vi "Locking_using_Photoacoustic_signal_usingcrorrected_intercept_2_custom_locking_with_runningavg_power.vi"() -> ()   [LabVIEW 2021]
uses:
  <vilib>/userDefined/High Color/IMAQdx.ctl
  <vilib>/Analysis/coordinate.llb/2D Cartesian Coordinate Rotation (Array).vi
  <vilib>/Analysis/6fits.llb/Confidence Interval (Linear).vi
  <vilib>/Instr/_visa.llb/VISA Configure Serial Port (Instr).vi
  <vilib>/Analysis/3filter.llb/Zero Phase Filter (DBL).vi
  <vilib>/Analysis/3filter.llb/Butterworth Filter (DBL).vi
  <vilib>/Utility/file.llb/Write Delimited Spreadsheet (DBL).vi
  <vilib>/vision/driver/NI_Vision_Acquisition_Software.lvlib
  <resource>/objmgr/imaqdx.rc
  <vilib>/Analysis/NI_AALBase.lvlib
  <vilib>/Analysis/NI_AAL_SigProc.lvlib
  <vilib>/Analysis/NI_AALPro.lvlib
  <vilib>/ptbypt/NI_PtbyPt.lvlib
  <vilib>/vision/NI_Vision_Development_Module.lvlib
  <instrlib>/Tektronix TBS 2000 Series/Tektronix TBS 2000 Series.lvlib
panel:
  out "Power normalized PAS CH1 2":dbl[](graph)
  out "mean 2":dbl format="%0.5f"
  out "PAS Mean":dbl format="%0.5f"
  out "Initaial value power":dbl format="%#_13g"
  out "mean":dbl format="%0.2f"
  out "millisecond timer value":u32
  in  "Avg Forpower meter":i32
  out "second pass wl 3":dbl format="%#_9g"
  in  "Number of Averages (16) 3":i32=8
  out "Number of Averages (16) 2":i32(ring)=8 items=["2"=2, "4"=4, "8"=8, "16"=16, "32"=32, "64"=64, "128"=128, "256"=256, "512"=512]
  in  "stop":bool
  out "PAS array":dbl[](array[numeric])
  in  "Running averaged power 2":bool
  out "Power(mJ) 2":dbl
  out "source 2":string
  out "Power Measurement with running average2":dbl[](graph)
  out "Normalized PAS 2":dbl format="%#_8g"
  out "Running avg power 2":dbl
  out "horzontal intercept 2":cluster{dbl[], dbl[]}(graph)
  out "Feedback sign 2":dbl
  out "Running avg power":dbl
  out "second pass wl 5":dbl format="%#_9g"
  out "PAS (Process value) 2":dbl format="%#_8g"
  in  "?":T1(tab)
  out "vertical Fringes 2":dbl[](graph)
  out "Horizontal Fringes 2":dbl[](graph)
  out "error out 11":errorcluster
  in  "thor wedge spacing 2":dbl=4.997771500000001 step=1e-06 format="%#_13g"
  out "known wavelength 2":dbl
  out "known wl 2":dbl[](array[numeric])=[591.188, 591.588, 591.988, 592.388, 592.788, 593.188]
  out "obseved wl 2":dbl[](array[numeric])=[591.1849, 591.5523, 591.984, 592.366, 592.7809, 593.169]
  out "Array 7":dbl[](array[numeric])
  out "error out 10":errorcluster
  out "Y Resolution 2":i32
  out "X Resolution 2":i32
  out "initila array horz. fringe 3":ext[](array[numeric])
  out "standard deviation 2":dbl format="%0.5f"
  out "observed wavelength 2":dbl
  out "horz.slope 3":dbl format="%#_7g"
  out "horz.intercept 2":dbl format="%#_8g"
  out "vert intercept 5":dbl
  out "vrt. slope 3":dbl format="%#_9g"
  out "x > y? 2":bool
  out "Locations 2":dbl[](array[numeric])
  in  "vert width 2":i32=5 min=3
  out "hor. std dev 2":dbl format="%0.5f"
  in  "horz. fringe width 2":i32=6 min=3
  in  "wedge angle of thor wedge 3":dbl=0.004681980000000043 format="%#_13g"
  in  "order 6":i32=1
  in  "order 5":i32=2
  out "d value 2":dbl format="%#_10e"
  out "vert.wl 2":dbl
  out "intercept 2":dbl
  out "vert wavelength 2":cluster{dbl[], dbl[]}(graph)
  out "horz intercept value 2":dbl[](array[numeric])
  out "Verticle slope":cluster{dbl[], dbl[]}(graph)
  in  "dimension size":i32=10
  in  "element 3":dbl=0.1 format="%#_15g"
  in  "dimension size 2":i32=10
  in  "element 2":dbl=0.1 format="%#_15g"
  out "vert inteer":dbl[](array[numeric])
  out "Loop time (ms) 2":u32
  out "Array 6":dbl[](array[numeric])
  out "Array 5":ext[](array[numeric])
  out "Buffer Number Out 2":u32
  in  "saturation 3":u32(slide) scale=0.0..128.0
  in  "Gain 3":u32(slide)=1 scale=1.0..128.0
  in  "exposure 3":ext(slide)=0.5 scale=0.0..0.5 scale format="%#_12g"
  out "EnumStrings[] 2":string[](array[string])
  in  "contrast 3":ext(slide)=0.5 scale=0.0..0.5 scale format="%#_12g"
  in  "camera property 2":bool
  in  "index 12":i32=90
  in  "length 11":i32=660
  in  "index 11":i32=400
  in  "length 10":i32=501
  out "horizontal fringe 3":dbl[][](graph)
  in  "index 10":i32=30
  in  "vert-vertical_array length":i32=850
  in  "index 9":i32=500
  in  "length 9":i32=1112
  in  "Slide":dbl(slide)=-2.6530612244897958
  out "VERT FRINGE":dbl[][](graph)
  out "x-y 2":ext
  in  "CONTRAST CUTT OFF VALUE":ext=0.015 format="%#_13g"
  out "initial array vert.  fringe 2":ext[](array[numeric])
  out "Meter":dbl(knob) scale=0.02..0.1 scale format="%#_4g"
  in  "Slide 4":dbl(slide)=-10.204081632653061
  out "count 3":dbl
  out "initial time 2":u32
  out "initial array vert 2":ext[](array[numeric])
  out "initial array horz 3":ext[](array[numeric])
  in  "Tab Control 2":enum32{"real time wavelength measurement"}(tab)
  out "Vertical intercept vs real time":cluster{dbl[], dbl[]}(graph)
  in  "image depth (bits) 4":string(combo)="8 bit" caption="image depth (bits)"
  in  "millisecond timer value 3":u16
  in  "stop 3":bool
  in  "Calibration 3":dbl=4.0
  in  "pixel size (nm) 4":dbl=4500.0 format="%#_13g"
  out "?":string
  out "error out 9":errorcluster
  out "error out 8":errorcluster
  out "INITIALtime":u32
  out "Boolean 3":bool
  out "element":dbl
  out "Power normalized PAS CH1":dbl[](graph)
  out "Power Measurement":dbl[](graph)
  out "Photo acoustic signal (PAS)":dbl[](graph)
  out "error out 7":cluster{"status":bool, "code":i32}
  in  "Source (1: Channel 2) 2":i32(ring)=2 items=["Math", "Channel 1", "Channel 2", "Channel 3", "Channel 4"]
  in  "Source (1: Channel 1)":i32(ring)=1 items=["Math", "Channel 1", "Channel 2", "Channel 3", "Channel 4"]
  in  "thor wedge spacing":dbl=4.997771500000001 step=1e-06 format="%#_13g"
  out "known wavelength":dbl
  in  "wedge spacing 2":dbl=0.8629192 step=1e-06 format="%#_13g"
  out "known wl":dbl[](array[numeric])=[591.188, 591.588, 591.988, 592.388, 592.788, 593.188]
  out "obseved wl":dbl[](array[numeric])=[591.1849, 591.5523, 591.984, 592.366, 592.7809, 593.169]
  in  "Calibration 2":dbl=4.0
  out "initial time":u32
  out "x/y 2":dbl
  in  "y":u32
  in  "Step size":i32=1
  out "Motor position":dbl format="%.12f"
  out "Measurement CH1":dbl
  out "Measurement CH2":dbl
  out "Numeric":i32
  in  "Number of steps":i32=10000
  in  "Measurement Slot (0: Immediate) 2":i32(ring) items=["Immediate", "Measurement 1", "Measurement 2", "Measurement 3", "Measurement 4", "Measurement 5", "Measurement 6"]
  in  "Measurement Slot (0: Immediate) 1":i32(ring)=1 items=["Immediate", "Measurement 1", "Measurement 2", "Measurement 3", "Measurement 4", "Measurement 5", "Measurement 6"]
  in  "Measurement Type (30: Rise)":i32(ring)=26 items=["Amplitude", "Area", "Burst", "Cycle Area", "Cycle Mean", "Cycle RMS", "Delay RR", "Delay RF", "Delay FR", "Delay FF", "Fall Time", "Frequency", "High Reference", "Low Reference", "Max", "Mean", "Min", "- Duty Cycle", "- Edge Count", "- Overshoot", "- Pulse Count", "- Width", "+ Duty Cycle", "+ Edge Count", "Period", "Phase", "Peak-to-Peak", "+ Overshoot", "+ Pulse Count", "+ Width", "Rise", "RMS"]
  out "GetPositionCounter":i32
  in  "Starting value":dbl=1.04067 format="%#.12f"
  out "Power(mJ)":dbl
  out "source":string
  out "stepcount":dbl[](array[numeric])
  in  "stop 2":bool
  out "CH1signal":dbl[](array[numeric])
  out "MesCH1":dbl
  in  "Manual scan step":dbl=5e-06
  in  "Manual scan in steps\n of":dbl=1e-06
  in  "Stepmulti[lPID":dbl=1e-07
  in  "Power":bool
  in  "Stop main loop":bool
  out "All channel 2":u16[](array[numeric])
  in  "Start scan":bool
  out "Oscilloscope Loop time":u32
  out "Boolean 2":bool
  in  "Acquisition Type (0:Sample)":i32(ring)=2 items=["Sample", "Peak Detect", "Average", "Hi Res"]
  in  "Number of Averages (16)":i32(ring)=8 items=["2"=2, "4"=4, "8"=8, "16"=16, "32"=32, "64"=64, "128"=128, "256"=256, "512"=512]
  out "new pressure":dbl
  in  "Array":dbl[](array[numeric])
  out "count":dbl
  out "vrt. slope":dbl format="%#_9g"
  out "initial array horz":ext[](array[numeric])
  out "initila array horz. fringe":ext[](array[numeric])
  in  "?":enum32{"Page 1"}(tab)
  in  "VISA for power supply 2":refnum<visa-resource-name>="COM10"
  out "read buffer 2":string
  in  "VISA resource name Power":refnum<visa-resource-name>="COM7"
  in  "VISA resource name Oscilliscope (TCPIP::10.10.7.221::INSTR)":refnum<visa-resource-name>="TCPIP::10.10.7.223::INSTR"
  out "RAW Image 2":T2(plugin-control)
  out "Wavelength vs time 2":cluster{dbl[], dbl[]}[](graph)
  out "?":string
  in  "?":T1(tab)
  in  "confidence level vert. fringe 2":dbl=0.65 format="%.2f"
  in  "threshold vert. fringe  2":dbl=7.0 format="%0.2f"
  in  "sampling freq. vert. fringe 2":dbl=1.0000000000000002 format="%0.2f"
  in  "calibration factor vert. fringe 4":dbl=12000.0
  in  "confidence level horz. fringe 2":dbl=0.65 format="%.2f"
  in  "sampling freq. horz. fringe 2":dbl=1.0 format="%0.2f"
  in  "threshold horz. fringe 2":dbl format="%0.2f"
  in  "calibration factor horz. fringe  2":dbl=2000.0
  in  "no. of average  2":i8=1
  in  "sample length 3":i32=10
  in  "wedge spacing 3":dbl=1.3793000000000004 step=1e-06 format="%#_13g"
  in  "wedge angle (rad) 3":dbl=0.008144042500000389 format="%#_13g"
  out "PAS (Process value)":dbl format="%#_8g"
  in  "Session In   3":T3="cam4"
  in  "Locking ON":bool
  in  "setpoint":dbl format="%.4f"
  out "Output (V) 2":dbl format="%.2f"
  out "Waveform Data from oscilloscope":T4(graph)
  in  "Delay Time (s)":dbl=1.0
  in  "Factor proportional":dbl
  out "Boolean":bool
  out "Read value":dbl
  in  "Set Transition  wavelength":dbl format="%#_10g"
  out "+ve":bool
  out "Normalized PAS":dbl format="%#_3g"
  out "?":string
  out "?":string
  in  "Manual voltage change":dbl
  out "Running averaged Power normalized PAS CH1 2":dbl[](graph)
  out "Running normalized PAS":dbl
  out "second pass wl 4":dbl format="%#_7g"
  out "?":string
  out "new tm":dbl
  # "Control parameter"
  # "First pass cal."
  # "second pass cal."
  # "First pass wavelength"
types:
  T1 = enum32{"vertical Fringes parameter", "Horizontal Fringes parameter"}
  T2 = typedef "IMAQ Image.ctl" = refnum<image>
  T3 = typedef "IMAQdx.ctl" = refnum<k21>
  T4 = cluster{"Initial X":dbl, "X Increment":dbl, "Waveform Array":dbl[]}[]
  T5 = typedef "Image Type" = u32
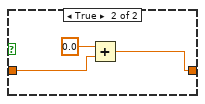
[diagram p8: hidden frame]
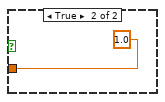
[diagram p12: hidden frame]
diagram:
  w5 = 0.0
  w23 = T5 4 items=["Grayscale (U8)", "Grayscale (I16)", "Grayscale (SGL)", "Complex (CSG)", "RGB (U32)", "HSL (U32)", "RGB (U64)", "Grayscale (U16)"] ("Image Type")
  w47 = T5 4 items=["Grayscale (U8)", "Grayscale (I16)", "Grayscale (SGL)", "Complex (CSG)", "RGB (U32)", "HSL (U32)", "RGB (U64)", "Grayscale (U16)"] ("Image Type")
  w70 = 0.0 ("count")
  n1 = Wait (ms)(milliseconds to wait="y") -> ()  [unwired: 1 out]
  n2 = Divide(x=u32 1000, y="y") -> (x/y=→"x/y 2":dbl)
  n3 = Tick Count (ms)() -> (millisecond timer value=→"initial time":u32)
  n4 = Tick Count (ms)() -> (millisecond timer value=→"initial time 2":u32)
  n5 = local write "new tm"(w70) -> ()
  n6 = call <instrlib>:"Initialize.vi"("Reset Device (True)"=FALSE ("Reset (True)"), "VISA resource name"="VISA resource name Oscilliscope (TCPIP::10.10.7.221::INSTR)") -> ("error out"=w55:errorcluster, "VISA resource name out"=w69:refnum<visa-resource-name>)  [unwired: 8 in]
  n7 = call <vilib>:"IMAQdx Open Camera.vi"("Session In"="Session In   3") -> ("error out"=w25:errorcluster, "Session Out"=w24:T3)  [unwired: 9 in]
  n8 = call "IMAQ Create"("Image Name"="256", "Image Type"=w23) -> ("New Image"=w20:T2, "error out"=→"error out 11":errorcluster)  [unwired: 3 in]
  n9 = call "IMAQ Create"("Image Name"="sau", "Image Type"=w47) -> ("New Image"=w45:T2, "error out"=→"error out 8":errorcluster)  [unwired: 3 in]
  n10 = call <vilib>:"IMAQdx Configure Grab.vi"("error in"=w25, "Session In"=w24) -> ("error out"=w44:errorcluster, "Session Out"=w50:T3)  [unwired: 8 in]
  n11 = call-poly "VISA Configure Serial Port"("VISA resource name"="VISA resource name Power", "baud rate (9600)"=u32 115200) -> ("VISA resource name out"=w56:refnum<visa-resource-name>)  [unwired: 12 in, 1 out]
  n12 = VISA Open(VISA resource name=w56) -> (VISA resource name=w6:refnum<visa-resource-name>)  [unwired: 4 in, 1 out]
  n13 = Initialize Array(w5, "Number of Averages (16) 3") -> (w4:dbl[])
  n14 = local write "initial array vert 2"(ext[] array[1280 elements] ("initial array vert")) -> ()
  n15 = local write "initial array vert.  fringe 2"(ext[] array[640 elements] ("initial array vert.  fringe")) -> ()
  n16 = local write "initial array horz"(ext[] array[1261 elements] ("initial array horz")) -> ()
  n17 = local write "initila array horz. fringe"(ext[] array[1261 elements] ("initila array horz. fringe")) -> ()
  n18 = local write "initial array vert.  fringe 2"(ext[] array[1280 elements] ("initial array")) -> ()
  n19 = Tick Count (ms)() -> (millisecond timer value=w53:u32)
  n20 = while {
    tunnel: w44 -> [w159]
    tunnel: w45 -> [w94]
    tunnel: w50 -> [w82]
    tunnel: [w128] -> w41
    shift-right: [w130] -> w17
    shift-left: i32[] [] -> [w152]
    shift-right: [w137] -> w10
    shift-left: dbl[] [] -> [w132]
    shift-right: [w124] -> w30
    shift-left: u32[] [] -> [w138]
    shift-right: [w125] -> w16
    shift-left: dbl[] [] -> [w126]
    shift-right: [w113] -> w15
    shift-left: dbl[] [] -> [w112]
    shift-right: [w110] -> _
    shift-left: dbl[] [] -> [w109]
    shift-right: [w75] -> _
    shift-left: dbl[] [] -> [w106]
    tunnel: w20 -> [w83]
    stop <- "stop 3" stop-if-true
    w84 = 5000 ("Timeout (ms)")
    n21 = local read "no. of average  2"() -> (w141:i8)
    n22 = Wait Until Next ms Multiple(millisecond multiple="millisecond timer value 3") -> ()  [unwired: 1 out]
    n23 = call <vilib>:"IMAQdx Grab2.vi"("Timeout (ms)"=w84, "Image In"=w83, "Session In"=w82) -> ("Image Out"=w77:T2)  [unwired: 5 in, 3 out]
    n24 = call <vilib>:"IMAQdx Grab2.vi"("Timeout (ms)"=w84, "error in"=w159, "Wait for Next Buffer? (Yes)"=FALSE, "Image In"=w94, "Session In"=w82) -> ("error out"=w97:errorcluster, "Buffer Number Out"=→"Buffer Number Out 2":u32, "Image Out"=w95:T2, "Session Out"=w129:T3)  [unwired: 3 in]
    "error out 10" <- w97
    "RAW Image 2" <- w95
    n25 = local read "count 3"() -> (w143:dbl)
    n26 = call "IMAQ Rotate"("error in (no error)"=w97, "Angle (degrees)"="Slide", "Image Dst"=w95, "Image Src"=w94) -> ("error out"=w96:errorcluster, "Image Dst Out"=w98:T2)  [unwired: 6 in]
    n27 = Add(x=w141, y=1.0) -> (x+y=w140:dbl)
    n28 = Greater Or Equal?(x=w143, y=w140) -> (x >= y?=w139:bool)
    n29 = call "IMAQ ColorImageToArray"("Image"=w98) -> ("Image Pixels (U32)"=w156:u32[][])  [unwired: 3 in, 2 out]
    n30 = call "IMAQ GetImageInfo"("Image"=w98) -> ("Y Resolution"=w154:i32, "X Resolution"=w153:i32)  [unwired: 3 in, 6 out]
    "Y Resolution 2" <- w154
    "X Resolution 2" <- w153
    n31 = case shown="True" w139 {
      frame False {
      }
      frame True {
        n32 = local write "count 3"(0.0 ("count")) -> ()
        n33 = local write "initial array vert.  fringe 2"(ext[] array[1280 elements] ("initial array")) -> ()
        n34 = local write "initial array horz 3"(ext[] array[1280 elements] ("initial array 2")) -> ()
        n35 = local write "initial array vert 2"(ext[] array[1282 elements] ("initial array vert")) -> ()
      }
    }
    n36 = call "IMAQ Rotate"("Angle (degrees)"="Slide 4", "Image Src"=w77) -> ("Image Dst Out"=w76:T2)  [unwired: 8 in, 1 out]
    n37 = Divide(x=w156, y=u32 4294967295) -> (x/y=w107:dbl[][])
    n38 = call "IMAQ ColorImageToArray"("Image"=w76) -> ("Image Pixels (U32)"=w81:u32[][])  [unwired: 3 in, 2 out]
    n39 = case shown="True" w139 {
      tunnel: [w205 w208] -> w124
      tunnel: w138 -> [w205 w206]
      frame False {
      }
      frame True {
        n40 = Tick Count (ms)() -> (millisecond timer value=w209:u32)
        n41 = local read "initial time 2"() -> (w213:u32)
        n42 = feedback #1() -> (w214:u32)  [unwired: 1 in]
        n43 = feedback-in #1(w209) -> ()
        n44 = Subtract(x=w209, y=w214) -> (x-y=→"Loop time (ms) 2":u32)
        n45 = Subtract(x=w209, y=w213) -> (x-y=w210:u32)
        n46 = Divide(x=w210, y=1000) -> (x/y=w207:dbl)
        n47 = Build Array (concatenate)(w206, w207) -> (w208:dbl[])
      }
    }
    "Array 6" <- w124
    n48 = Divide(x=w81, y=u32 4294967295) -> (x/y=w79:dbl[][])
    n49 = call-poly <vilib>:"2D Cartesian Coordinate Rotation.vi"() -> ()  [unwired: 9 in, 3 out]
    n50 = Wait (ms)(milliseconds to wait=u32 400) -> ()  [unwired: 1 out]
    n51 = Array Subset(array=w79, index (row)="index 12", length (row)="length 11", index (col)="index 11", length (col)="length 10") -> (w120:dbl[][])
    "horizontal fringe 3" <- w120
    n52 = for {
      tunnel: [w440] -> w147 mode=indexing
      tunnel: w120 -> [w439] mode=indexing
      n53 = Add Array Elements(numeric array=w439) -> (sum=w440:dbl)
    }
    n54 = case shown="True" "camera property 2" {
      tunnel: w96 -> [w182 w184]
      tunnel: w129 -> [w183 w185]
      tunnel: [w183 w194] -> w128
      tunnel: [w182 w192] -> _
      frame False {
      }
      frame True {
        n55 = property class="IMAQdx"(reference=w185, error in=w184, "ActiveAttribute"="CameraAttributes::Saturation::Value", "ValueU32"="saturation 3") -> (reference out=w197:T3, error out=w198:errorcluster)
        n56 = property class="IMAQdx"(reference=w197, error in=w198, "ActiveAttribute"="CameraAttributes::Gain::Value", "ValueU32"="Gain 3") -> (reference out=w202:T3, error out=w201:errorcluster)
        n57 = property class="IMAQdx"(reference=w202, error in=w201, "ActiveAttribute"="CameraAttributes::Exposure::Value", "ValueDBL"="exposure 3") -> (reference out=w191:T3, error out=w187:errorcluster)
        n58 = property class="IMAQdx"(reference=w191, error in=w187, "ActiveAttribute"="CameraAttributes::Contrast::Value", "ValueDBL"="contrast 3") -> (reference out=w190:T3, error out=w186:errorcluster)
        n59 = property class="IMAQdx"(reference=w190, error in=w186) -> (reference out=w194:T3, error out=w192:errorcluster, "EnumStrings[]"=→"EnumStrings[] 2":string[])
      }
    }
    n60 = Array Subset(array=w107, index (row)="index 10", length (row)="vert-vertical_array length", index (col)="index 9", length (col)="length 9") -> (w115:dbl[][])
    n61 = Transpose 2D Array(2D array=w115) -> (transposed array=w93:dbl[][])
    "VERT FRINGE" <- w93
    n62 = for {
      tunnel: [w442] -> w151 mode=indexing
      tunnel: w93 -> [w441] mode=indexing
      n63 = Add Array Elements(numeric array=w441) -> (sum=w442:dbl)
    }
    n64 = local read "image depth (bits) 4"() -> (w133:string)
    n65 = Fract/Exp String To Number(string="image depth (bits) 4") -> ()  [unwired: 3 in, 2 out]
    n66 = Fract/Exp String To Number(string=w133) -> (number=w134:dbl)  [unwired: 3 in, 1 out]
    n67 = Divide(x=w151, y=w154) -> (x/y=w150:dbl[])
    n68 = Scale By Power Of 2(n=i16 12, x=ext 1.0) -> (x*2^n=w148:ext)
    n69 = Divide(x=w147, y=w153) -> (x/y=w146:dbl[])
    n70 = Multiply(x=w150, y=w148) -> (x*y=w114:ext[])
    n71 = Scale By Power Of 2(n=w134, x=ext 1.0) -> (x*2^n=w144:ext)
    n72 = Multiply(x=w146, y=w144) -> (x*y=→"initila array horz. fringe 3":ext[])
    n73 = Reverse 1D Array(array=w114) -> (reversed array=→"initial array vert.  fringe 2":ext[])
    n74 = local read "initial array vert.  fringe 2"() -> (w91:ext[])
    n75 = Array Subset(array=w91, index=100, length=20) -> (w90:ext[])
    n76 = local read "no. of average  2"() -> (w136:i8)
    n77 = Array Max & Min(array=w90) -> (max value=w89:ext, min value=w88:ext)  [unwired: 2 out]
    n78 = Subtract(x=w89, y=w88) -> (x-y=w85:ext)
    "x-y 2" <- w85
    "Meter" <- w85
    n79 = Greater Or Equal?(x=w85, y="CONTRAST CUTT OFF VALUE") -> (x >= y?=w87:bool)
    n80 = case shown="True" w87 {
      tunnel: [_ w163] -> w104
      tunnel: [_ w162] -> w102
      tunnel: [_ w161] -> w92
      frame False {
      }
      frame True {
        n81 = local read "no. of average  2"() -> (w165:i8)
        n82 = for {
          N: "no. of average  2" -> [_]
          tunnel: [w179] -> w163
          tunnel: [w174] -> w161
          tunnel: [w171] -> w164
          stop <- w171 stop-if-true
          n83 = local read "initial array vert.  fringe 2"() -> (w181:ext[])
          n84 = local read "no. of average  2"() -> (w172:i8)
          n85 = local read "initial array vert 2"() -> (w180:ext[])
          n86 = local read "count 3"() -> (w173:dbl)
          n87 = local read "no. of average  2"() -> (w178:i8)
          n88 = Add(x=w180, y=w181) -> (x+y=w179:ext[])
          n89 = Not Equal?(x=w173, y=w172) -> (x != y?=w171:bool)
          n90 = local read "count 3"() -> (w177:dbl)
          n91 = local read "count 3"() -> (w176:dbl)
          n92 = local write "initial array vert 2"(w179) -> ()
          n93 = Increment(x=w176) -> (x+1=w175:dbl)
          n94 = Equal?(x=w177, y=w178) -> (x = y?=w174:bool)
          n95 = local write "count 3"(w175) -> ()
        }
        n96 = for {
          N: w165 -> [_]
          tunnel: [w170] -> w162
          tunnel: w164 -> [w167]
          stop <- w167 stop-if-true
          n97 = local read "initila array horz. fringe 3"() -> (w168:ext[])
          n98 = local read "initial array horz 3"() -> (w169:ext[])
          n99 = Add(x=w169, y=w168) -> (x+y=w170:ext[])
          n100 = local write "initial array horz 3"(w170) -> ()
        }
      }
    }
    "Array 5" <- w102
    n101 = case shown="True" w92 {
      tunnel: [w223 w327] -> w130
      tunnel: w152 -> [w223 w354]
      tunnel: w102 -> [_ w352]
      tunnel: w104 -> [_ w351]
      tunnel: w124 -> [_ w332]
      tunnel: [w224 w274] -> w137
      tunnel: w124 -> [_ w243]
      tunnel: w136 -> [_ w331]
      tunnel: w132 -> [w224 w328]
      tunnel: [w222 w272] -> w125
      tunnel: w126 -> [w222 w275]
      tunnel: w124 -> [_ w273]
      tunnel: [w221 w250] -> w113
      tunnel: w112 -> [w221 w251]
      tunnel: w109 -> [w220 w248]
      tunnel: [w220 w247] -> w110
      tunnel: w106 -> [w219 w242]
      tunnel: [w219 w239] -> w75
      frame False {
      }
      frame True {
        n102 = local read "Calibration 3"() -> (w294:dbl)
        n103 = local read "pixel size (nm) 4"() -> (w292:dbl)
        n104 = Divide(x=w352, y=w331) -> (x/y=w230:ext[])
        n105 = local read "vrt. slope 3"() -> (w299:dbl)
        n106 = local read "no. of average  2"() -> (w353:i8)
        n107 = local read "wedge angle (rad) 3"() -> (w295:dbl)
        n108 = Divide(x=w351, y=w353) -> (x/y=w233:ext[])
        n109 = Initialize Array("element 2", "dimension size 2") -> (w236:dbl[])
        n110 = Initialize Array("element 3", "dimension size") -> (w232:dbl[])
        n111 = local read "second pass wl 3"() -> (w297:dbl)
        n112 = Multiply(x=w292, y=w294) -> (x*y=w293:dbl)
        n113 = Multiply(x=w299, y=w293) -> (x*y=w298:dbl)
        n114 = Multiply(x=w295, y=w298) -> (x*y=w296:dbl)
        "observed wavelength 2" <- w296
        n115 = call-poly <vilib>:"Zero Phase Filter.vi"("Forward Coefficients"=w236, "X"=w233) -> ()  [unwired: 8 in, 2 out]
        n116 = call-poly <vilib>:"Butterworth Filter.vi"("order"="order 6", "sampling freq: fs"="sampling freq. vert. fringe 2", "X"=w233) -> ("Filtered X"=w231:dbl[])  [unwired: 5 in, 1 out]
        n117 = call-poly <vilib>:"Zero Phase Filter.vi"("Forward Coefficients"=w232, "Reverse Coefficients"=w232) -> ()  [unwired: 8 in, 2 out]
        n118 = local read "second pass wl 4"() -> (w276:dbl)
        n119 = Array Size(array=w231) -> (size(s)=w280:i32)
        n120 = Build Array (concatenate)(w328, w297) -> (w274:dbl[])
        n121 = Bundle(w332, w274) -> (w270:cluster{dbl[], dbl[]})  [unwired: 1 in]
        n122 = Format Into String(format string="wavelength: %5.3f nm", w296) -> (resulting string=→"?":string)  [unwired: 2 in, 1 out]
        n123 = call-poly <vilib>:"Butterworth Filter.vi"("order"="order 5", "sampling freq: fs"="sampling freq. horz. fringe 2", "X"=w230) -> ("Filtered X"=w229:dbl[])  [unwired: 5 in, 1 out]
        n124 = Array Size(array=w229) -> (size(s)=w283:i32)
        n125 = Build Array (concatenate)(w275, w276) -> (w272:dbl[])
        n126 = Bundle(w273, w272) -> (w271:cluster{dbl[], dbl[]})  [unwired: 1 in]
        n127 = Subtract(x=w280, y=50) -> (x-y=w278:i32)
        n128 = Subtract(x=w283, y=10) -> (x-y=w282:i32)
        n129 = Build Array(w271, w270) -> (→"Wavelength vs time 2":cluster{dbl[], dbl[]}[])
        n130 = Array Subset(array=w229, index=10, length=w282) -> (w263:dbl[])
        "Horizontal Fringes 2" <- w263
        n131 = Array Subset(array=w231, index=30, length=w278) -> (w253:dbl[])
        "vertical Fringes 2" <- w253
        n132 = call <vilib>:"Peak Detector.vi"("peaks/valleys"=enum32{"Peaks", "Valleys"}."Valleys", "width"="horz. fringe width 2", "threshold"="threshold horz. fringe 2", "X"=w263) -> ("Locations"=w323:dbl[])  [unwired: 3 in, 4 out]
        n133 = call <vilib>:"Peak Detector.vi"("peaks/valleys"=enum32{"Peaks", "Valleys"}."Peaks", "width"="horz. fringe width 2", "X"=w263) -> ("Locations"=w322:dbl[])  [unwired: 4 in, 4 out]
        n134 = call <vilib>:"Peak Detector.vi"("peaks/valleys"=enum32{"Peaks", "Valleys"}."Valleys", "width"="vert width 2", "threshold"="threshold vert. fringe  2", "X"=w253) -> ("Locations"=w309:dbl[])  [unwired: 3 in, 4 out]
        "Locations 2" <- w309
        n135 = call <vilib>:"Peak Detector.vi"("peaks/valleys"=enum32{"Peaks", "Valleys"}."Peaks", "width"="vert width 2", "X"=w253) -> ("Locations"=w302:dbl[])  [unwired: 4 in, 4 out]
        n136 = local read "Calibration 3"() -> (w259:dbl)
        n137 = local read "pixel size (nm) 4"() -> (w260:dbl)
        n138 = Build Array (concatenate)(w323, w322) -> (w321:dbl[])
        n139 = Index Array(array=w302, index=0) -> (element=w305:dbl)
        n140 = Build Array (concatenate)(w309, w302) -> (w347:dbl[])
        n141 = Sort 1D Array(array=w321) -> (sorted array=w318:dbl[])
        n142 = Array Size(array=w318) -> (size(s)=w320:i32)
        n143 = Index Array(array=w309, index=0) -> (element=w306:dbl)
        n144 = local read "wedge angle of thor wedge 3"() -> (w255:dbl)
        n145 = Sort 1D Array(array=w347) -> (sorted array=w345:dbl[])
        n146 = Array Size(array=w345) -> (size(s)=w346:i32)
        n147 = Multiply(x=w260, y=w259) -> (x*y=w257:dbl)
        n148 = Greater?(x=w306, y=w305) -> (0:w304:bool)
        "x > y? 2" <- w304
        n149 = local read "horz.slope 3"() -> (w258:dbl)
        n150 = for {
          N: w346 -> [_]
          tunnel: [w438] -> w344 mode=concatenating
          i -> [w437]
          n151 = Build Array(w437) -> (w438:i32[])
        }
        n152 = for {
          N: w320 -> [_]
          tunnel: [w364] -> w319 mode=concatenating
          i -> [w363]
          n153 = Build Array(w363) -> (w364:i32[])
        }
        n154 = Multiply(x=w258, y=w257) -> (x*y=w256:dbl)
        n155 = call <vilib>:"Linear Fit.vi"("Y"=w318, "X"=w319) -> ("slope"=w314:dbl, "intercept"=w252:dbl)  [unwired: 9 in, 3 out]
        "horz.slope 3" <- w314
        "horz.intercept 2" <- w252
        n156 = Build Array (concatenate)(w251, w252) -> (w250:dbl[])
        "horz intercept value 2" <- w250
        n157 = Multiply(x=w256, y=w255) -> (x*y=w249:dbl)
        "vert.wl 2" <- w249
        n158 = call <vilib>:"Linear Fit.vi"("Y"=w345, "X"=w344) -> ("slope"=w241:dbl, "intercept"=w310:dbl)  [unwired: 9 in, 3 out]
        "vrt. slope 3" <- w241
        "intercept 2" <- w310
        n159 = Build Array (concatenate)(w248, w249) -> (w247:dbl[])
        n160 = case shown="False" w304 {
          tunnel: w310 -> [w357 w362]
          tunnel: [w359 w361] -> w254
          frame False {
            n161 = local read "vrt. slope 3"() -> (w358:dbl)
            n162 = Add(x=w357, y=0.0) -> (x+y=w356:dbl)
            n163 = Add(x=w358, y=w356) -> (x+y=w359:dbl)
          }
          frame True {
            n164 = Add(x=0.0, y=w362) -> (x+y=w361:dbl)
          }
        }
        "vert intercept 5" <- w254
        n165 = call-poly <vilib>:"Linear Fit Intervals.vi"("Y"=w318, "confidence level"="confidence level horz. fringe 2", "X"=w319, "slope"=w314, "intercept"=w252) -> ("delta slope"=w286:dbl)  [unwired: 6 in, 4 out]
        n166 = call-poly <vilib>:"Linear Fit Intervals.vi"("Y"=w345, "confidence level"="confidence level vert. fringe 2", "X"=w344, "slope"=w241, "intercept"=w310) -> ("delta slope"=w340:dbl)  [unwired: 6 in, 4 out]
        n167 = local read "horz intercept value 2"() -> (w245:dbl[])
        n168 = Bundle(w243, w247) -> (→"vert wavelength 2":cluster{dbl[], dbl[]})  [unwired: 1 in]
        n169 = Bundle(w243, "horz intercept value 2"=w245) -> (→"horzontal intercept 2":cluster{dbl[], "horz intercept value 2":dbl[]})  [unwired: 1 in]
        n170 = Divide(x=w340, y=w241) -> (x/y=w338:dbl)
        n171 = local read "sample length 3"() -> (w277:i32)
        n172 = local read "sample length 3"() -> (w288:i32)
        n173 = local read "vrt. slope 3"() -> (w268:dbl)
        n174 = Divide(x=w286, y=w314) -> (x/y=w312:dbl)
        n175 = call <vilib>:"Standard Deviation PtByPt.vi"("x"=w254, "sample length"=w277) -> ("standard deviation"=w333:dbl)  [unwired: 1 in, 2 out]
        "standard deviation 2" <- w333
        n176 = Multiply(x=w268, y=9.0) -> (x*y=w266:dbl)
        n177 = Multiply(x=w312, y=1000000.0) -> (x*y=w311:dbl)
        n178 = Multiply(x=w338, y=1000000.0) -> (x*y=w337:dbl)
        n179 = Multiply(x=w266, y=1e-06) -> (x*y=→"d value 2":dbl)
        n180 = Format Into String(format string="horz. fringe slope error: %5.2f ppm", w311) -> (resulting string=→"?":string)  [unwired: 2 in, 1 out]
        n181 = Build Array (concatenate)(w354, w254) -> (w327:dbl[])
        "vert inteer" <- w327
        n182 = Bundle(w243, w327) -> (→"Vertical intercept vs real time":cluster{dbl[], dbl[]})  [unwired: 1 in]
        n183 = Format Into String(format string="vert. fringe slope error: %5.2f ppm", w337) -> (resulting string=→"?":string)  [unwired: 2 in, 1 out]
        n184 = call <vilib>:"Standard Deviation PtByPt.vi"("x"=w252, "sample length"=w288) -> ("standard deviation"=w291:dbl)  [unwired: 1 in, 2 out]
        "hor. std dev 2" <- w291
        n185 = Multiply(x=w333, y="calibration factor vert. fringe 4") -> (x*y=w334:dbl)
        n186 = Build Array (concatenate)(w242, w241) -> (w239:dbl[])
        n187 = Format Into String(format string="wavelength sens vert fringe: %5.2f MHz", w334) -> (resulting string=→"?":string)  [unwired: 2 in, 1 out]
        n188 = Multiply(x=w291, y="calibration factor horz. fringe  2") -> (x*y=w290:dbl)
        n189 = Bundle(w243, w239) -> (→"Verticle slope":cluster{dbl[], dbl[]})  [unwired: 1 in]
        n190 = Format Into String(format string="wavelength sens horz fri: %5.2f MHz", w290) -> (resulting string=→"?":string)  [unwired: 2 in, 1 out]
        n191 = flat-sequence {
          frame #0 {
            (unwired) 632.807 ("x")
            (unwired) 802.0
            n192 = local read "observed wavelength 2"() -> (w365:dbl)
            n193 = local read "wedge spacing 3"() -> (w369:dbl)
            n194 = local read "vert intercept 5"() -> (w368:dbl)
            n195 = local read "pixel size (nm) 4"() -> (w371:dbl)
            n196 = Multiply(x=4.0, y=w369) -> (x*y=w398:dbl)
            n197 = Multiply(x=4.0, y=w368) -> (x*y=w394:dbl)
            n198 = Multiply(x=1000000.0, y=w398) -> (x*y=w397:dbl)
            n199 = Multiply(x=2.0, y=w368) -> (x*y=w383:dbl)
            n200 = Multiply(x=2.0, y=w369) -> (x*y=w388:dbl)
            n201 = Multiply(x="pixel size (nm) 4", y=w394) -> (x*y=w392:dbl)
            n202 = local read "wedge angle (rad) 3"() -> (w370:dbl)
            n203 = Multiply(x=w371, y=w383) -> (x*y=w380:dbl)
            n204 = local read "wedge angle (rad) 3"() -> (w366:dbl)
            n205 = Multiply(x=1000000.0, y=w388) -> (x*y=w384:dbl)
            n206 = Tangent(1:w370) -> (0:w393:dbl)
            n207 = Tangent(1:w366) -> (0:w381:dbl)
            n208 = Multiply(x=w381, y=w380) -> (x*y=w376:dbl)
            n209 = Multiply(x=w393, y=w392) -> (x*y=w391:dbl)
            n210 = Add(x=w384, y=w376) -> (x+y=w375:dbl)
            n211 = Divide(x=w375, y=w365) -> (x/y=w379:dbl)
            n212 = Add(x=w391, y=w397) -> (x+y=w386:dbl)
            n213 = Subtract(x=w379, y=0.5) -> (x-y=w377:dbl)
            n214 = Round To Nearest(number=w377) -> (nearest integer value=w373:dbl)
            n215 = Multiply(x=2.0, y=w373) -> (x*y=w372:dbl)
            n216 = Add(x=w372, y=1.0 ("x")) -> (x+y=w385:dbl)
            n217 = Divide(x=w386, y=w385) -> (x/y=→"second pass wl 3":dbl)
          }
          frame #1 {
            n218 = local read "thor wedge spacing 2"() -> (w434:dbl)
            n219 = local read "horz.intercept 2"() -> (w435:dbl)
            n220 = local read "second pass wl 3"() -> (w405:dbl)
            n221 = local read "pixel size (nm) 4"() -> (w433:dbl)
            n222 = local read "pixel size (nm) 4"() -> (w406:dbl)
            n223 = Multiply(x=4.0, y=w434) -> (x*y=w408:dbl)
            n224 = Multiply(x=4.0, y=w435) -> (x*y=w411:dbl)
            n225 = local read "wedge angle of thor wedge 3"() -> (w404:dbl)
            n226 = Multiply(x=1000000.0, y=w408) -> (x*y=w409:dbl)
            n227 = Multiply(x=2.0, y=w435) -> (x*y=w421:dbl)
            n228 = Multiply(x=2.0, y=w434) -> (x*y=w416:dbl)
            n229 = Multiply(x=w406, y=w411) -> (x*y=w413:dbl)
            n230 = local read "wedge angle of thor wedge 3"() -> (w403:dbl)
            n231 = Multiply(x=w433, y=w421) -> (x*y=w424:dbl)
            n232 = Multiply(x=1000000.0, y=w416) -> (x*y=w420:dbl)
            n233 = Tangent(1:w403) -> (0:w412:dbl)
            n234 = Tangent(1:w404) -> (0:w423:dbl)
            n235 = Multiply(x=w423, y=w424) -> (x*y=w428:dbl)
            n236 = Multiply(x=w412, y=w413) -> (x*y=w414:dbl)
            n237 = Add(x=w420, y=w428) -> (x+y=w429:dbl)
            n238 = Divide(x=w429, y=w405) -> (x/y=w425:dbl)
            n239 = Add(x=w414, y=w409) -> (x+y=w418:dbl)
            n240 = Subtract(x=w425, y=0.5) -> (x-y=w427:dbl)
            n241 = Round To Nearest(number=w427) -> (nearest integer value=w431:dbl)
            n242 = Multiply(x=2.0, y=w431) -> (x*y=w432:dbl)
            n243 = Add(x=w432, y=1.0 ("x")) -> (x+y=w419:dbl)
            n244 = Divide(x=w418, y=w419) -> (x/y=→"second pass wl 4":dbl)
          }
        }
      }
    }
  }
  "Array 7" <- w30
  n245 = local write "initial array horz 3"(ext[] array[1280 elements] ("initial array 2")) -> ()
  n246 = while {
    shift-right: [w475] -> w66
    shift-left: w69 -> [w455]
    shift-right: [w474] -> w65
    shift-left: w55 -> [w454]
    tunnel: i32[] [] -> [w463]
    tunnel: "Source (1: Channel 1)" -> [w457]
    tunnel: "Source (1: Channel 2) 2" -> [w456]
    tunnel: w6 -> [w451]
    tunnel: "Avg Forpower meter" -> [w448]
    shift-right: [w447] -> _
    shift-left: w4 -> [w446]
    shift-right: [w444] -> _
    shift-left: w5 -> [w445]
    stop <- "Stop main loop" stop-if-true
    n247 = Build Array(w457, w456) -> (w476:i32[])
    "All channel 2" <- w476
    n248 = feedback #2(u32 0 ("millisecond timer value")) -> (w471:u32)
    n249 = Tick Count (ms)() -> (millisecond timer value=w470:u32)
    n250 = feedback-in #2(w470) -> ()
    n251 = Subtract(x=w470, y=w471) -> (x-y=→"Oscilloscope Loop time":u32)
    n252 = call <instrlib>:"Configure Acquisition.vi"("error in (no error)"=w454, "Number of Averages (16)"="Number of Averages (16)", "Acquisition Type (0:Sample)"="Acquisition Type (0:Sample)", "VISA resource name"=w455) -> ("error out"=w460:errorcluster, "VISA resource name out"=w461:refnum<visa-resource-name>)  [unwired: 6 in]
    n253 = call <instrlib>:"Read Multiple Waveforms.vi"("error in (no error)"=w460, "Sources"=w476, "VISA resource name"=w461) -> ("error out"=w472:errorcluster, "Waveform Graph"=→"Waveform Data from oscilloscope":T4, "VISA resource name out"=w473:refnum<visa-resource-name>)  [unwired: 6 in]
    n254 = case shown="True" "Start scan" {
      tunnel: w473 -> [w480 w505]
      tunnel: w472 -> [w479 w504]
      tunnel: [w480 w500] -> w475
      tunnel: [w479 w499] -> w474
      tunnel: dbl[] [] -> [_ w496]
      tunnel: dbl[] [] -> [_ w495]
      tunnel: dbl[] [] -> [_ w494]
      tunnel: dbl[] [] -> [_ w493]
      tunnel: w463 -> [_ w492]
      tunnel: dbl[] [] -> [_ w490]
      tunnel: w451 -> [_ w489]
      tunnel: "Start scan" -> [_ w488]
      tunnel: dbl[] [] -> [_ w487]
      tunnel: w448 -> [_ w486]
      tunnel: w446 -> [w478 w485]
      tunnel: [w478 w484] -> w447
      tunnel: w445 -> [w477 w483]
      tunnel: [w477 w482] -> w444
      tunnel: dbl[] [] -> [_ w481]
      frame False {
      }
      frame True {
        n255 = flat-sequence {
          tunnel: w505 -> [w528]
          tunnel: w504 -> [w527]
          tunnel: w496 -> [w526]
          tunnel: w494 -> [_]
          tunnel: w493 -> [_]
          tunnel: w495 -> [w524]
          tunnel: [w523] -> w500
          tunnel: [w522] -> w499
          tunnel: [w521] -> w497
          tunnel: w492 -> [w520]
          tunnel: [w519] -> w491
          tunnel: [w525] -> w498
          tunnel: w490 -> [w515]
          tunnel: w489 -> [w514]
          tunnel: w488 -> [w513]
          tunnel: w487 -> [w512]
          tunnel: w486 -> [w511]
          tunnel: w485 -> [w510]
          tunnel: [w509] -> w484
          tunnel: w483 -> [w508]
          tunnel: [w507] -> w482
          tunnel: w481 -> [w506]
          frame #0 {
            n256 = local write "Measurement CH1"(0.0 ("Measurement CH1")) -> ()
            n257 = local write "Measurement CH2"(0.0 ("Measurement CH2")) -> ()
            n258 = local read "Starting value"() -> (w516:dbl)
            n259 = local write "Motor position"(w516) -> ()
            n260 = while {
              tunnel: w527 -> [w597]
              tunnel: w528 -> [w595]
              shift-right: [w565] -> w525
              shift-left: w526 -> [w562]
              shift-right: [w591] -> w521
              shift-left: w524 -> [w602]
              tunnel: [w585] -> w523
              tunnel: [w583] -> w522
              shift-right: [w589] -> w519
              shift-left: w520 -> [w590]
              shift-right: [w571] -> _
              shift-left: w515 -> [w572]
              tunnel: w514 -> [w570]
              tunnel: w513 -> [_]
              shift-right: [w553] -> _
              shift-left: w512 -> [w561]
              tunnel: w511 -> [w559]
              tunnel: w510 -> [w558]
              tunnel: [w557] -> w509
              tunnel: w508 -> [w555]
              tunnel: [w554] -> w507
              shift-right: [w530] -> _
              shift-left: w506 -> [w531]
              i -> [w556]
              stop <- "stop 2" stop-if-true
              (unwired) 10000 ("waitTimeout")
              # "1 step = 0.056 GHz"
              # "Step"
              # "CH2"
              # "CH1"
              n261 = call-poly "VISA Configure Serial Port"("VISA resource name"="VISA for power supply 2", "baud rate (9600)"=u32 9600, "data bits (8)"=u16 8, "parity (0:none)"=enum16{"None", "Odd", "Even", "Mark", "Space"}."None") -> ("VISA resource name out"=w547:refnum<visa-resource-name>, "error out"=w546:errorcluster)  [unwired: 5 in, 5 out]
              n262 = local read "Motor position"() -> (w573:dbl)
              n263 = VISA Write(VISA resource name=w547, write buffer=":MEASure:VOLTage?\n" ("Command"), error in (no error)=w546) -> (VISA resource name out=w545:refnum<visa-resource-name>, error out=w544:errorcluster)  [unwired: 1 out]
              n264 = local read "All channel 2"() -> (w593:u16[])
              n265 = flat-sequence {
                tunnel: w544 -> [w605]
                tunnel: [w605] -> w549
                tunnel: w545 -> [w604]
                tunnel: [w604] -> w548
                tunnel: u32 200 ("delay before read (ms)") -> [w606]
                frame #0 {
                  n266 = Wait (ms)(milliseconds to wait=w606) -> ()  [unwired: 1 out]
                }
              }
              n267 = local read "Measurement CH1"() -> (w529:dbl)
              "MesCH1" <- w529
              "mean 2" <- w529
              n268 = local read "Measurement CH2"() -> (w599:dbl)
              n269 = property class="Instr"(reference=w548, error in=w549) -> (reference out=w535:refnum<visa-resource-name>, error out=w550:errorcluster, "Serial Settings:Number of Bytes at Serial Port"=w551:u32)
              n270 = Multiply(x=w573, y=0.056) -> (x*y=w575:dbl)
              n271 = call <instrlib>:"Read Multiple Waveforms.vi"("error in (no error)"=w597, "Sources"=w593, "VISA resource name"=w595) -> ("error out"=w596:errorcluster, "Waveform Graph"=w592:T4, "VISA resource name out"=w594:refnum<visa-resource-name>)  [unwired: 6 in]
              n272 = local write "Waveform Data from oscilloscope"(w592) -> ()
              n273 = Divide(x=w575, y=30.0) -> ()  [unwired: 1 out]
              n274 = Build Array (concatenate)(w562, w529) -> (w565:dbl[])
              "CH1signal" <- w565
              n275 = Build Array (concatenate)(w602, w599) -> (w591:dbl[])
              n276 = Build Array (concatenate)(w590, w573) -> (w589:dbl[])
              "stepcount" <- w589
              n277 = VISA Read(VISA resource name=w535, byte count=w551, error in (no error)=w550) -> (VISA resource name out=w536:refnum<visa-resource-name>, read buffer=w537:string)  [unwired: 2 out]
              n278 = case shown="True" "Locking ON" {
                tunnel: w537 -> [_ w608]
                tunnel: w536 -> [_ w607]
                frame False {
                }
                frame True {
                  n279 = local read "PAS (Process value)"() -> (w611:dbl)
                  n280 = Greater?(x="setpoint", y=w611) -> (0:w609:bool)
                  "Boolean" <- w609
                  n281 = case shown="True" w609 {
                    tunnel: w608 -> [_ w615]
                    tunnel: w607 -> [_ w614]
                    frame False {
                    }
                    frame True {
                      n282 = Fract/Exp String To Number(string=w615) -> (number=w621:dbl)  [unwired: 3 in, 1 out]
                      "Read value" <- w621
                      n283 = Wait Until Next ms Multiple(millisecond multiple=u32 10) -> ()  [unwired: 1 out]
                      n284 = local read "second pass wl 4"() -> (w619:dbl)
                      n285 = Greater?(x=w619, y="Set Transition  wavelength") -> (0:w617:bool)
                      "+ve" <- w617
                      n286 = call "RIGOL_power_supply(SubVI).vi"("Delay Time (s)"="Delay Time (s)", "voltage_in 3"="Manual voltage change", "VISA Refnum in"=w614) -> ()  [unwired: 7 in, 2 out]
                      n287 = case shown="False" w617 {
                        tunnel: [1.0 ("Feedback sign") 1.0 ("Feedback sign")] -> w616
                        frame False {
                          # "in false use -1"
                        }
                        frame True {
                        }
                      }
                      "Feedback sign 2" <- w616
                      n288 = Multiply(x="Factor proportional", y=w616) -> (x*y=w622:dbl)
                      n289 = Add(x=w621, y=w622) -> (x+y=→"Output (V) 2":dbl)
                      "read buffer 2" <- w615
                    }
                  }
                }
              }
              n290 = local read "Source (1: Channel 1)"() -> (w578:i32)
              n291 = Bundle(w589, w591) -> (w598:cluster{dbl[], dbl[]})  [unwired: 1 in]
              n292 = Bundle(w589, w565) -> (w603:cluster{dbl[], dbl[]})  [unwired: 1 in]
              n293 = local read "Source (1: Channel 2) 2"() -> (w577:i32)
              n294 = Build Array(w603, w598) -> ()  [unwired: 1 out]
              n295 = call <instrlib>:"Configure Measurement.vi"("VISA resource name"=w594, "Measurement Slot (0: Immediate)"="Measurement Slot (0: Immediate) 1", "Measurement Source 1 (1: Channel 1)"=w578, "Measurement Type (30: Rise)"="Measurement Type (30: Rise)", "error in (no error)"=w596) -> ("VISA resource name out"=w600:refnum<visa-resource-name>, "error out"=w601:errorcluster)  [unwired: 9 in]
              n296 = Array Size(array=w565) -> (size(s)=w566:i32)
              n297 = call <instrlib>:"Configure Measurement.vi"("VISA resource name"=w600, "Measurement Slot (0: Immediate)"="Measurement Slot (0: Immediate) 2", "Measurement Source 1 (1: Channel 1)"=w577, "Measurement Type (30: Rise)"="Measurement Type (30: Rise)", "error in (no error)"=w601) -> ("VISA resource name out"=w588:refnum<visa-resource-name>, "error out"=w587:errorcluster)  [unwired: 9 in]
              n298 = Index Array(array=w565, index=w566) -> (element=w560:dbl)
              "element" <- w560
              n299 = call <instrlib>:"Read Waveform Measurement.vi"("error in (no error)"=w587, "Measurement Slot (0: Immediate)"="Measurement Slot (0: Immediate) 1", "VISA resource name"=w588) -> ("error out"=w584:errorcluster, "Measurement"=w534:dbl, "VISA resource name out"=w586:refnum<visa-resource-name>)  [unwired: 6 in]
              "Measurement CH1" <- w534
              n300 = Less?(x=w560, y=5000.0) -> (x < y?=w564:bool)
              "Boolean 3" <- w564
              n301 = call <instrlib>:"Read Waveform Measurement.vi"("error in (no error)"=w584, "Measurement Slot (0: Immediate)"="Measurement Slot (0: Immediate) 2", "VISA resource name"=w586) -> ("error out"=w583:errorcluster, "Measurement"=→"Measurement CH2":dbl, "VISA resource name out"=w585:refnum<visa-resource-name>)  [unwired: 6 in]
              n302 = case shown="True" w564 {
                tunnel: w529 -> [_ w630]
                tunnel: w562 -> [w627 _]
                tunnel: w561 -> [_ w635]
                tunnel: [w627 w634] -> w553
                frame False {
                }
                frame True {
                  n303 = call <vilib>:"Mean PtByPt.vi"("x"=w630, "sample length"=10) -> ("mean"=w629:dbl)  [unwired: 2 in, 1 out]
                  n304 = Build Array (concatenate)(w635, w629) -> (w634:dbl[])
                  "Photo acoustic signal (PAS)" <- w634
                  "PAS array" <- w634
                  n305 = Array Size(array=w634) -> (size(s)=w637:i32)
                  n306 = Decrement(x=w637) -> (x-1=w636:i32)
                  n307 = Index Array(array=w634, index=w636) -> (element=w633:dbl)
                  n308 = Multiply(x=w633, y=1.0) -> (x*y=→"PAS (Process value)":dbl)
                }
              }
              n309 = case shown="True" "Power" {
                tunnel: w570 -> [w642 w675]
                tunnel: [w642 w674] -> _
                tunnel: [w641 w650] -> w571
                tunnel: w572 -> [w641 w667]
                tunnel: w553 -> [_ w666]
                tunnel: w556 -> [_ w656]
                tunnel: w559 -> [_ w655]
                tunnel: w558 -> [w640 w654]
                tunnel: [w640 w653] -> w557
                tunnel: w555 -> [w639 w652]
                tunnel: [w639 w651] -> w554
                tunnel: w531 -> [w638 w645]
                tunnel: [w638 w643] -> w530
                frame False {
                }
                frame True {
                  # "Power measurement"
                  n310 = VISA Write(VISA resource name=w675, write buffer="*CVU") -> (VISA resource name out=w673:refnum<visa-resource-name>)  [unwired: 1 in, 2 out]
                  n311 = VISA Read(VISA resource name=w673, byte count=u32 25) -> (VISA resource name out=w674:refnum<visa-resource-name>, read buffer=w670:string)  [unwired: 1 in, 2 out]
                  n312 = Fract/Exp String To Number(string=w670) -> (number=w669:dbl)  [unwired: 3 in, 1 out]
                  n313 = Multiply(x=w669, y=1000.0) -> (x*y=w648:dbl)
                  "Power(mJ)" <- w648
                  n314 = call <vilib>:"Mean PtByPt.vi"("x"=w648, "sample length"=10) -> ("mean"=w647:dbl)  [unwired: 2 in, 1 out]
                  n315 = Build Array (concatenate)(w667, w647) -> (w650:dbl[])
                  "Power Measurement" <- w650
                  n316 = Increment(x=w656) -> (x+1=w662:i32)
                  n317 = Quotient & Remainder(x=w656, y=w655) -> (x-y*floor(x/y)=w659:i32)  [unwired: 1 out]
                  n318 = Index Array(array=w654, index=w659) -> (element=w657:dbl)
                  n319 = Less?(x=w655, y=w662) -> (x < y?=w660:bool)
                  n320 = Subtract(x=w652, y=w657) -> (x-y=w658:dbl)
                  n321 = Select(t=w655, s=w660, f=w662) -> (s? t:f=w661:i32)
                  n322 = Replace Array Subset(array=w654, new element=w648, index=w659) -> (w653:dbl[])
                  n323 = Add(x=w648, y=w658) -> (x+y=w651:dbl)
                  n324 = Divide(x=w651, y=w661) -> (x/y=→"Running avg power":dbl)
                  n325 = Divide(x=w666, y=w650) -> (x/y=w663:dbl[])
                  "Power normalized PAS CH1" <- w663
                  n326 = Array Size(array=w663) -> (size(s)=w664:i32)
                  n327 = Decrement(x=w664) -> (x-1=w665:i32)
                  n328 = Index Array(array=w663, index=w665) -> (element=w644:dbl)
                  "Normalized PAS" <- w644
                  n329 = Build Array (concatenate)(w645, w644) -> (w643:dbl[])
                  "Power normalized PAS CH1 2" <- w643
                }
              }
              n330 = call <vilib>:"Mean PtByPt.vi"("x"=w534, "sample length"=10) -> ("mean"=→"PAS Mean":dbl)  [unwired: 2 in, 1 out]
              "Numeric" <- "Number of steps"
            }
          }
        }
        n331 = Build Array(w491, w498, w497) -> (w501:dbl[][])
        n332 = Transpose 2D Array(2D array=w501) -> (transposed array=w502:dbl[][])
        n333 = call-poly <vilib>:"Write Delimited Spreadsheet.vi"("format (%.3f)"="  %.3f", "2D data"=w502) -> ()  [unwired: 12 in, 2 out]
      }
    }
    "Boolean 2" <- "Start scan"
    "Number of Averages (16) 2" <- "Number of Averages (16)"
  }
  n334 = Divide(x=w53, y=1000.0) -> (x/y=→"INITIALtime":dbl)
  n335 = local write "initial array vert 2"(ext[] array[960 elements] ("initial array vert")) -> ()
  n336 = local write "initial array vert.  fringe 2"(ext[] array[1280 elements] ("initial array")) -> ()
  n337 = local write "initial array horz 3"(ext[] array[1280 elements] ("initial array 2")) -> ()
  n338 = while {
    tunnel: "Number of Averages (16) 3" -> [w685]
    tunnel: w6 -> [w682]
    shift-right: [w681] -> _
    shift-left: dbl[] [] -> [w684]
    shift-right: [w678] -> _
    shift-left: w4 -> [w679]
    shift-right: [w677] -> _
    shift-left: w5 -> [w680]
    i -> [w686]
    stop <- "stop" stop-if-true
    n339 = case shown="True" "Running averaged power 2" {
      tunnel: w682 -> [w690 w731]
      tunnel: [w690 w730] -> _
      tunnel: [w689 w707] -> w681
      tunnel: w684 -> [w689 w723]
      tunnel: w686 -> [_ w713]
      tunnel: w685 -> [_ w712]
      tunnel: w679 -> [w688 w711]
      tunnel: [w688 w710] -> w678
      tunnel: w680 -> [w687 w709]
      tunnel: [w687 w708] -> w677
      frame False {
      }
      frame True {
        # "Power measurement"
        n340 = local read "initial time 2"() -> (w697:u32)
        n341 = Tick Count (ms)() -> (millisecond timer value=w696:u32)
        n342 = VISA Write(VISA resource name=w731, write buffer="*CVU") -> (VISA resource name out=w729:refnum<visa-resource-name>)  [unwired: 1 in, 2 out]
        n343 = Subtract(x=w697, y=w696) -> (x-y=w695:u32)
        n344 = Multiply(x=w695, y=0.001) -> (x*y=→"millisecond timer value":dbl)
        n345 = VISA Read(VISA resource name=w729, byte count=u32 25) -> (VISA resource name out=w730:refnum<visa-resource-name>, read buffer=w726:string)  [unwired: 1 in, 2 out]
        n346 = Fract/Exp String To Number(string=w726) -> (number=w725:dbl)  [unwired: 3 in, 1 out]
        n347 = Multiply(x=w725, y=1000.0) -> (x*y=w694:dbl)
        "Power(mJ) 2" <- w694
        n348 = call <vilib>:"Mean PtByPt.vi"() -> ()  [unwired: 4 in, 2 out]
        n349 = call <vilib>:"Mean PtByPt.vi"("x"=w694, "sample length"=8) -> ("mean"=w692:dbl)  [unwired: 2 in, 1 out]
        "mean" <- w692
        n350 = Build Array (concatenate)(w723, w692) -> (w707:dbl[])
        "Power Measurement with running average2" <- w707
        n351 = Increment(x=w713) -> (x+1=w719:i32)
        n352 = Quotient & Remainder(x=w713, y=w712) -> (x-y*floor(x/y)=w716:i32)  [unwired: 1 out]
        n353 = Wait Until Next ms Multiple(millisecond multiple=u32 100) -> ()  [unwired: 1 out]
        n354 = Index Array(array=w711, index=w716) -> (element=w714:dbl)
        n355 = Less?(x=w712, y=w719) -> (x < y?=w717:bool)
        n356 = Subtract(x=w709, y=w714) -> (x-y=w715:dbl)
        n357 = Select(t=w712, s=w717, f=w719) -> (s? t:f=w718:i32)
        n358 = Replace Array Subset(array=w711, new element=w694, index=w716) -> (w710:dbl[])
        n359 = Add(x=w694, y=w715) -> (x+y=w708:dbl)
        n360 = Divide(x=w708, y=w718) -> (x/y=→"Running avg power 2":dbl)
        n361 = for {
          N: 8 -> [_]
          n362 = local read "Initaial value power"() -> (w733:dbl)
          n363 = local read "Power(mJ) 2"() -> (w734:dbl)
          n364 = Add(x=w734, y=w733) -> (x+y=w732:dbl)
          n365 = local write "Initaial value power"(w732) -> ()
        }
        n366 = local read "PAS array"() -> (w706:dbl[])
        n367 = Divide(x=w706, y=w707) -> (x/y=w702:dbl[])
        "Running averaged Power normalized PAS CH1 2" <- w702
        n368 = Array Size(array=w702) -> (size(s)=w720:i32)
        n369 = Decrement(x=w720) -> (x-1=w721:i32)
        n370 = Index Array(array=w702, index=w721) -> (element=→"Normalized PAS 2":dbl)
        n371 = Array Size(array=w702) -> (size(s)=w704:i32)
        n372 = Decrement(x=w704) -> (x-1=w703:i32)
        n373 = Index Array(array=w702, index=w703) -> (element=→"Running normalized PAS":dbl)
      }
    }
  }
  n374 = local write "Boolean 2"(FALSE ("Boolean")) -> ()
  n375 = call <instrlib>:"Close.vi"("error in (no error)"=w65, "VISA resource name"=w66) -> ()  [unwired: 9 in, 1 out]
  n376 = call <vilib>:"IMAQdx Close Camera.vi"("Session In"=w41) -> ("error out"=w12:errorcluster)  [unwired: 10 in]
  n377 = Build Array(w17, w16, w10, w15) -> (w14:dbl[][])
  n378 = Transpose 2D Array(2D array=w14) -> (transposed array=w13:dbl[][])
  n379 = call-poly <vilib>:"Write Delimited Spreadsheet.vi"("format (%.3f)"="%.5f", "2D data"=w13, "append to file? (new file:F)"=FALSE ("append to file? (F)"), "error in (no error)"=w12) -> ("error out"=→"error out 9":errorcluster)  [unwired: 10 in, 1 out]
  "count" <- 0.0 ("count")
  "new tm" <- w70
  "new pressure" <- w70
  "initial array horz 3" <- ext[] array[960 elements] ("initial array horz")
  "initial array vert 2" <- ext[] array[1280 elements] ("initial array vert")
  "Initaial value power" <- 0.0 ("Numeric 2")
